vi "ep_Sliding Reference Voltage.vi"(0 "voltage RMS (1/2) (1 cycle)":T1(array[cluster]), 1 "restart (F)":bool, 5 "nominal voltage [V]":dbl=230.0, 7 "type of reference voltage":enum16{"Constant", "Sliding"}(ring), 9 "voltage flags":bool[](array[boolean]), 11 "error in (no error)":errorcluster) -> (4 "reference voltages":dbl[](array[numeric]), 15 "error out":errorcluster)   [LabVIEW 2014, in "NI_EP_Power Quality.lvlib"]
doc: "This VI returns constant or sliding reference voltages for each phase."
uses:
  <vilib>/addons/Electrical Power/PQ/NI_EP_Power Quality.lvlib
  <vilib>/Analysis/5stat.llb/RMS (DBL).vi
  <vilib>/Analysis/NI_AALPro.lvlib
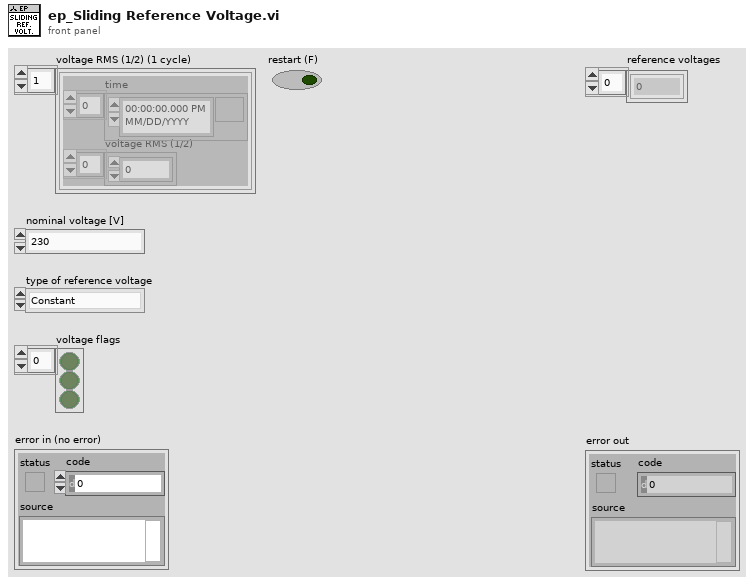
[diagram p1: front panel]
types:
  T1 = cluster{"time":timestamp[], "voltage RMS (1/2)":dbl[]}[]
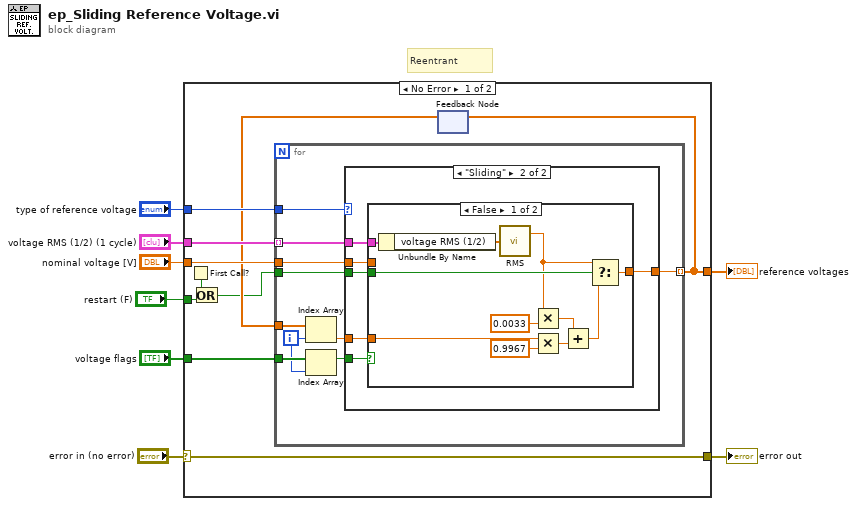
[diagram p0: block diagram]
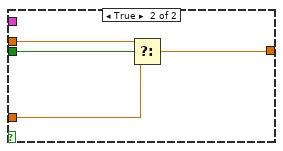
[diagram p3: hidden frame]
diagram:
  # "Reentrant"
  n1 = case shown="No Error" "error in (no error)" {
    selector: "error in (no error)" -> [w9 w51]
    tunnel: "voltage RMS (1/2) (1 cycle)" -> [w18 _]
    tunnel: "type of reference voltage" -> [w17 _]
    tunnel: "nominal voltage [V]" -> [w16 _]
    tunnel: "voltage flags" -> [w15 _]
    tunnel: [w14 _] -> w4
    tunnel: "restart (F)" -> [w12 _]
    tunnel: [w9 w51] -> w1
    frame No Error {
      n2 = First Call?() -> (First Call?: T/F=w11:bool)
      n3 = Or(x=w11, y=w12) -> (x .or. y?=w10:bool)
      n4 = feedback #1() -> (w13:dbl[])  [unwired: 1 in]
      n5 = for {
        tunnel: w18 -> [w25] mode=indexing
        tunnel: w17 -> [w28]
        tunnel: [w27] -> w14 mode=indexing
        tunnel: w16 -> [w26]
        tunnel: w15 -> [w21]
        tunnel: w13 -> [w23]
        tunnel: w10 -> [w24]
        i -> [w19]
        n6 = Index Array(array=w23, index=w19) -> (element=w22:dbl)
        n7 = Index Array(array=w21, index=w19) -> (element=w20:bool)
        n8 = case shown="\"Sliding\"" w28 {
          tunnel: [w29 w35] -> w27
          tunnel: w26 -> [w29 w31]
          tunnel: w25 -> [_ w33]
          tunnel: w22 -> [_ w30]
          tunnel: w24 -> [_ w32]
          tunnel: w20 -> [_ w34]
          frame "Constant", Default {
          }
          frame "Sliding" {
            n9 = case shown="False" w34 {
              tunnel: w33 -> [w46 _]
              tunnel: [w38 w47] -> w35
              tunnel: w30 -> [w41 w48]
              tunnel: w32 -> [w39 w50]
              tunnel: w31 -> [_ w49]
              frame False {
                n10 = Unbundle By Name(w46) -> ("voltage RMS (1/2)"=w45:dbl[])
                n11 = call-poly <vilib>:"RMS.vi"("X"=w45) -> ("rms value"=w37:dbl)  [unwired: 1 out]
                n12 = Multiply(x=w37, y=0.0033) -> (x*y=w43:dbl)
                n13 = Multiply(x=w41, y=0.9967) -> (x*y=w40:dbl)
                n14 = Add(x=w43, y=w40) -> (x+y=w36:dbl)
                n15 = Select(t=w37, s=w39, f=w36) -> (s? t:f=w38:dbl)
              }
              frame True {
                n16 = Select(t=w49, s=w50, f=w48) -> (s? t:f=w47:dbl)
              }
            }
          }
        }
      }
      n17 = feedback-in #1(w14) -> ()
    }
    frame Error {
    }
  }
  "reference voltages" <- w4
  "error out" <- w1
